vi "new NOT Filter.vi"(7 "a":refnum<class "Filter.lvclass">) -> (8 "not a":refnum<class "Filter.lvclass">)   [LabVIEW 2016, in "NOT Filter.lvclass"]
uses:
  NOT Filter.lvclass
  Filter Parent/Filter.lvclass
  C:/github/VeriStand-FPGA-Resource-Manager/Source/Client/Test CD/FPGA RM Test Client/Source/System Explorer/Filters/Filter Parent/Filter.lvclass
  NOT Filter.lvclass/NOT Filter.ctl
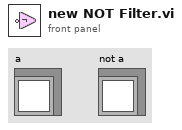
[diagram p1: front panel]
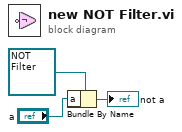
[diagram p0: block diagram]
diagram:
  n1 = Bundle By Name(cluster=refnum<class "NOT Filter.lvclass"> refnum ("NOT Filter in"), "a"="a") -> (→"not a":refnum<class "NOT Filter.lvclass">)
